vi "disable_by_name.vi"(8 "error in (no error)":errorcluster caption="错误输入（无错误）", 10 "name":string, 11 "MotorSystem 输入":refnum<class "MotorSystem.lvclass">) -> (0 "error out":errorcluster caption="错误输出", 3 "MotorSystem 输出":refnum<class "MotorSystem.lvclass">)   [LabVIEW 2016, in "MotionControl_UFO_3DOF.lvlib" / "MotorSystem.lvclass"]
uses:
  <userlib>/MotionControl_UFO_3DOF/MotorSystem/MotorSystem.lvclass
  <userlib>/MotionControl_UFO_3DOF/MotorSystem/MotorSystem.lvclass/MotorSystem.ctl
  <userlib>/MotionControl_UFO_3DOF/OneMotion/OneMotion.lvclass
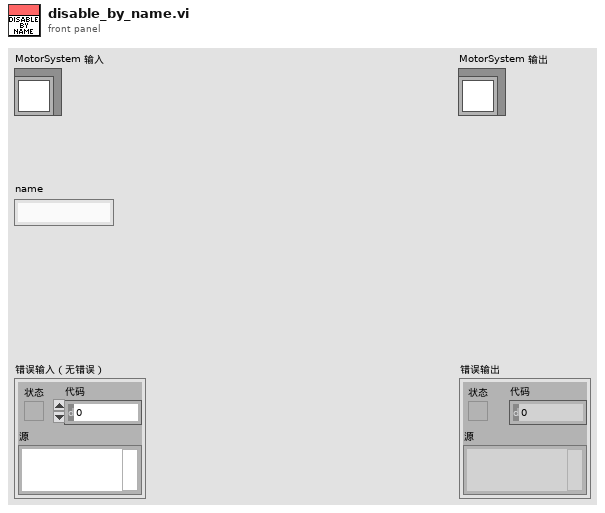
[diagram p1: front panel]
types:
  T1 = typedef "MotionControl_UFO_3DOF.lvlib/MotorSystem.lvclass/MotionCluster.ctl" = cluster{"OneMotion.lvclass":refnum<class "OneMotion.lvclass">, "connected?":bool, "default enabled?":bool, "enabled?":bool}
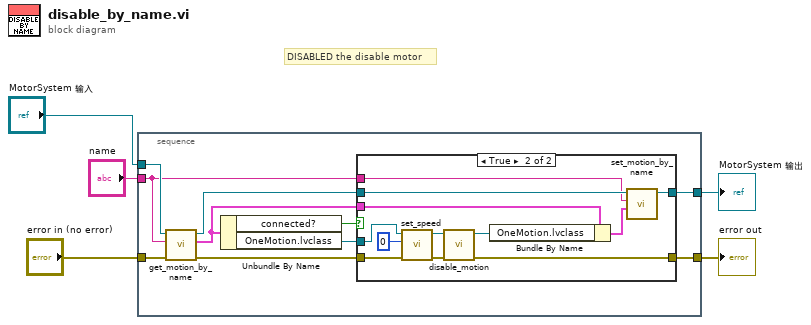
[diagram p0: block diagram]
diagram:
  # "DISABLED the disable motor"
  n1 = stacked-sequence {
    tunnel: [w14] -> w5
    tunnel: [w11] -> w3
    tunnel: "MotorSystem 输入" -> [w13]
    tunnel: "error in (no error)" -> [w15]
    tunnel: "name" -> [w10]
    frame #0 {
      n2 = call <userlib>:"get_motion_by_name.vi"("error in (no error)"=w15, "name"=w10, "MotorSystem in"=w13) -> ("error out"=w7:errorcluster, "motion cluster"=w9:T1, "MotorSystem out"=w12:refnum<class "MotorSystem.lvclass">)  [unwired: 6 in]
      n3 = Unbundle By Name(w9) -> ("connected?"=w6:bool, "OneMotion.lvclass"=w8:refnum<class "OneMotion.lvclass">)
      n4 = case shown="True" w6 {
        tunnel: [w16 w29] -> w14
        tunnel: w12 -> [w17 w28]
        tunnel: [w17 w27] -> w11
        tunnel: w10 -> [_ w26]
        tunnel: w9 -> [_ w25]
        tunnel: w8 -> [_ w22]
        tunnel: w7 -> [w16 w19]
        frame False {
        }
        frame True {
          n5 = call-dynamic "set_speed.vi"("error in (no error)"=w19, "speed"=0, "OneMotion 输入"=w22) -> ("error out"=w18:errorcluster, "OneMotion 输出"=w20:refnum<class "OneMotion.lvclass">)  [unwired: 7 in]
          n6 = call <userlib>:"disable_motion.vi"("error in (no error)"=w18, "OneMotion 输入"=w20) -> ("error out"=w29:errorcluster, "OneMotion 输出"=w24:refnum<class "OneMotion.lvclass">)  [unwired: 8 in]
          n7 = Bundle By Name(cluster=w25, "OneMotion.lvclass"=w24) -> (w23:T1)
          n8 = call <userlib>:"set_motion_by_name.vi"("簇"=w23, "name"=w26, "MotorSystem输入"=w28) -> ("MotorSystem输出"=w27:refnum<class "MotorSystem.lvclass">)  [unwired: 7 in, 1 out]
        }
      }
    }
  }
  "error out" <- w5
  "MotorSystem 输出" <- w3
